vi "Create_Rect.vi"(8 "error in (no error)":errorcluster caption="错误输入（无错误）", 9 "宽度":dbl, 10 "长度":dbl, 11 "矩形类 输入":refnum<class "矩形.lvclass"> caption="DNL_LabVIEW Object in") -> (0 "error out":errorcluster caption="错误输出", 3 "矩形类 输出":refnum<class "矩形.lvclass"> caption="DNL_LabVIEW Object out")   [LabVIEW 2013, in "矩形.lvclass"]
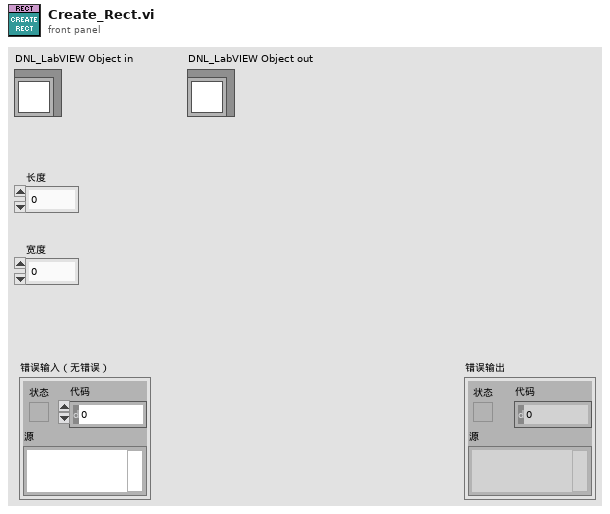
[diagram p1: front panel]
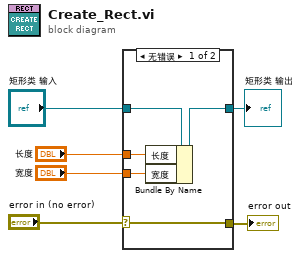
[diagram p0: block diagram]
diagram:
  n1 = case shown="无错误" "error in (no error)" {
    selector: "error in (no error)" -> [w10 w13]
    tunnel: [w10 w13] -> w5
    tunnel: [w9 w12] -> w3
    tunnel: "矩形类 输入" -> [w11 w12]
    tunnel: "长度" -> [w8 _]
    tunnel: "宽度" -> [w7 _]
    frame No Error {
      n2 = Bundle By Name(cluster=w11, "长度"=w8, "宽度"=w7) -> (w9:refnum<class "矩形.lvclass">)
    }
    frame Error {
    }
  }
  "error out" <- w5
  "矩形类 输出" <- w3
